vi "Controller_API_Init.vi"(8 "error in (no error)":errorcluster, 11 "Data in":T1={"Cmd"=enum."PrintChart", "Temperature"=0.0, "Logs"=""}) -> (0 "error out":errorcluster)   [LabVIEW 2020]
uses:
  #typedef_Controller_Data.ctl
  #typedef_ControllerQueue_States.ctl
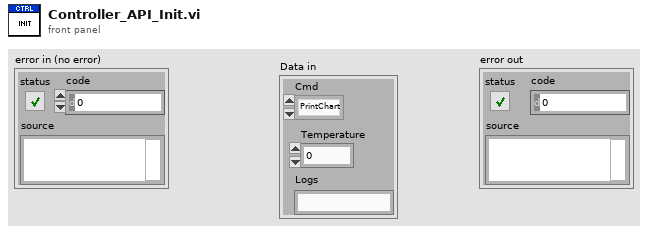
[diagram p1: front panel]
types:
  T1 = typedef "#typedef_Controller_Data.ctl" = cluster{"Cmd":enum16{"Idle", "PrintChart", "SendToDB", "Exit"}, "Temperature":dbl, "Logs":string}
  T2 = typedef "#typedef_ControllerQueue_States.ctl" = enum16{"Obtain", "GetRef", "Enqueue", "EnqueueAtOpp", "GetStatus", "Flush", "Release"}
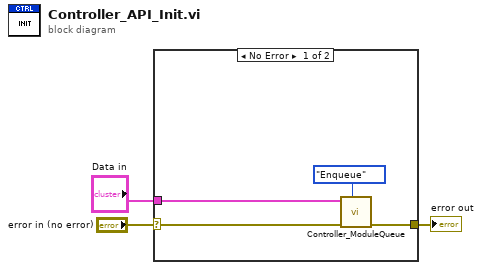
[diagram p0: block diagram]
diagram:
  n1 = case shown="No Error" "error in (no error)" {
    selector: "error in (no error)" -> [w6 w8]
    tunnel: [w5 w8] -> w2
    tunnel: "Data in" -> [w4 _]
    frame No Error {
      n2 = call "Controller_ModuleQueue.vi"(7:#typedef_ControllerQueue_States."Enqueue", "error in (no error)"=w6, "Data in"=w4) -> ("error out"=w5:errorcluster)  [unwired: 6 in, 2 out]
    }
    frame Error {
    }
  }
  "error out" <- w2
